vi "Untitled 5 (SubVI).vi"(4 "spleetbreedte\n      (mm)":dbl, 5 "Numeric 2":dbl, 6 "collimator afstand\n       (mm)":dbl, 7 "Numeric 6":dbl, 9 "Numeric":dbl, 10 "Numeric 7":dbl, 11 "fraction core\nannihilations":dbl) -> (0 "Numeric 3":dbl, 1 "Numeric 4":dbl, 2 "Numeric 5":dbl, 3 "Numeric 8":dbl)   [LabVIEW 2013]
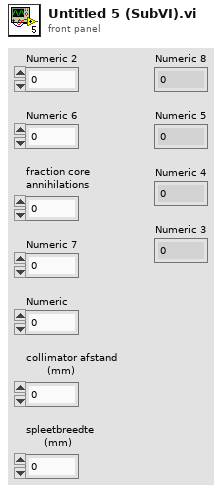
[diagram p1: front panel]
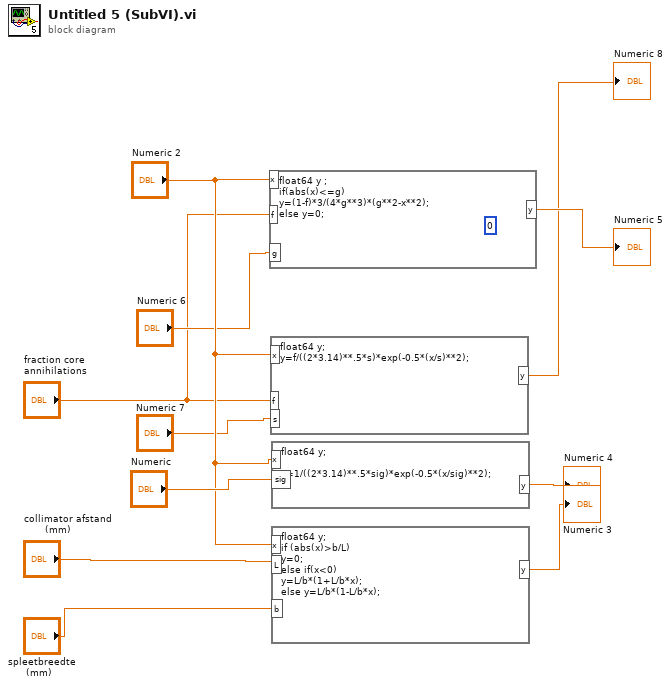
[diagram p0: block diagram]
diagram:
  (unwired) 0
  # "gauss"
  # "parabool"
  # "tentfunctie"
  n1 = formula code="float64 y ;\nif(abs(x)<=g)\ny=(1-f)*3/(4*g**3)*(g**2-x**2);\nelse y=0;"("x"="Numeric 2", "g"="Numeric 6", "f"="fraction core\nannihilations") -> ("y"=→"Numeric 5":dbl)
  n2 = formula code="float64 y;\ny=f/((2*3.14)**.5*s)*exp(-0.5*(x/s)**2);"("x"="Numeric 2", "s"="Numeric 7", "f"="fraction core\nannihilations") -> ("y"=→"Numeric 8":dbl)
  n3 = formula code="float64 y;\n\ny=1/((2*3.14)**.5*sig)*exp(-0.5*(x/sig)**2);"("x"="Numeric 2", "sig"="Numeric") -> ("y"=→"Numeric 4":dbl)
  n4 = formula code="float64 y;\nif (abs(x)>b/L)\ny=0;\nelse if(x<0)\ny=L/b*(1+L/b*x);\nelse y=L/b*(1-L/b*x);"("x"="Numeric 2", "b"="spleetbreedte\n      (mm)", "L"="collimator afstand\n       (mm)") -> ("y"=→"Numeric 3":dbl)
